vi "NMRvmefull6.vi"() -> ()   [LabVIEW 2013]
uses:
  <vilib>/Utility/file.llb/Read From Spreadsheet File (DBL).vi
  <vilib>/Analysis/NI_AALBase.lvlib
panel:
  out "Telnet error out":errorcluster
  in  "Real/quad Q curve":bool=TRUE
  out "Temperature (C)":dbl(graph)=14.38
  out "+3V supply":dbl=3.03 format="%_4g"
  out "Temp (C)":dbl=14.38 format="%_4g"
  in  "RemovePed":bool=TRUE
  in  "IF / LOG Det":bool
  in  "Q curve file":string="realback213.txt"
  out "File name 2":string="C:\\users\\plm\\Desktop\\rssmt\\realback213.txt"
  in  "AutoBaseline":bool=TRUE
  out "RF OK":bool=TRUE
  out "Peak area (V-MHz)":sgl=0.047433283 format="%.5f"
  in  "Gauss Fit":bool=TRUE
  out "NMR Graph + Fit":cluster{cluster{dbl, "Numeric":dbl}[]}[](graph)=[{[{212.6, "Numeric"=-0.014353571428571417}, {212.60999999999999, "Numeric"=0.00969880952378703}, {212.62, "Numeric"=0.006451190476215146}, {212.63, "Numeric"=0.01930357142857405}, {212.64, "Numeric"=0.0034559523809340603}, {212.65, "Numeric"=0.0017083333333586803}, {212.66, "Numeric"=0.004160714285719118}, {212.67, "Numeric"=-0.02268690476191927}, {212.68, "Numeric"=-0.002834523809498196}, {212.69, "Numeric"=-0.01118214285713618}, {212.7, "Numeric"=0.0006702380952269132}, {212.71, "Numeric"=-0.01337738095235555}, {212.72, "Numeric"=-0.006324999999991986}, {212.73, "Numeric"=-0.0047726190476272586}, {212.74, "Numeric"=-0.0005202380952584774}, {212.75, "Numeric"=-0.0027678571428481173}, {212.76, "Numeric"=-0.009515476190481851}, {212.77, "Numeric"=0.004936904761888499}, {212.78, "Numeric"=-0.01361071428570466}, {212.79, "Numeric"=0.009441666666663164}, {212.8, "Numeric"=-0.0016059523809648993}, {212.81, "Numeric"=0.009946428571438355}, {212.82, "Numeric"=0.011698809523807772}, {212.82999999999998, "Numeric"=0.009451190476178262}, {212.84, "Numeric"=0.0005035714285809706}, {212.85, "Numeric"=-0.013844047619048054}, {212.85999999999999, "Numeric"=0.004308333333324003}, {212.87, "Numeric"=-0.007039285714276826}, {212.88, "Numeric"=0.0008130952380957287}, {212.89, "Numeric"=0.0021654761904693603}, {212.9, "Numeric"=0.007617857142864972}, {212.91, "Numeric"=0.018070238095239086}, {212.92, "Numeric"=0.014822619047614286}, {212.93, "Numeric"=0.03257500000000636}, {212.94, "Numeric"=0.043427380952382036}, {212.95, "Numeric"=0.07847976190475882}, {212.96, "Numeric"=0.12533214285714733}, {212.97, "Numeric"=0.26208452380952457}, {212.98, "Numeric"=0.46923690476190294}, {212.99, "Numeric"=0.47378928571428536}, {213.0, "Numeric"=0.36984166666666674}, {213.01, "Numeric"=0.31639404761904666}, {213.02, "Numeric"=0.28634642857143067}, {213.03, "Numeric"=0.24109880952380847}, {213.04, "Numeric"=0.2555511904761899}, {213.05, "Numeric"=0.2537035714285755}, {213.06, "Numeric"=0.2389559523809498}, {213.07, "Numeric"=0.24110833333333284}, {213.08, "Numeric"=0.20696071428571997}, {213.09, "Numeric"=0.1666130952380907}, {213.1, "Numeric"=0.1359654761904753}, {213.11, "Numeric"=0.105517857142864}, {213.12, "Numeric"=0.0838702380952312}, {213.13, "Numeric"=0.08352261904761737}, {213.14000000000001, "Numeric"=0.06727500000000765}, {213.15, "Numeric"=0.060527380952371285}, {213.16, "Numeric"=0.05027976190475904}, {213.17000000000002, "Numeric"=0.06763214285715088}, {213.18, "Numeric"=0.056484523809510974}, {213.19, "Numeric"=0.010836904761900301}, {213.2, "Numeric"=0.019789285714290707}, {213.21, "Numeric"=-0.0011583333333497411}, {213.22, "Numeric"=0.002394047619041117}, {213.23, "Numeric"=-0.0070535714285668814}, {213.24, "Numeric"=-0.01370119047617081}, {213.25, "Numeric"=-0.01564880952381845}, {213.26, "Numeric"=-0.012996428571424894}, {213.27, "Numeric"=0.002355952380972765}, {213.28, "Numeric"=-0.0036916666666784066}, {213.29, "Numeric"=-0.00803928571428332}, {213.3, "Numeric"=-0.021786904761884066}, {213.31, "Numeric"=-0.007334523809538827}, {213.32, "Numeric"=-0.014282142857142105}, {213.33, "Numeric"=-0.0075297619047413195}, {213.34, "Numeric"=-0.00247738095239957}, {213.35, "Numeric"=-0.01902500000000132}, {213.36, "Numeric"=0.002227380952401034}, {213.37, "Numeric"=-0.0088202380952608}, {213.38, "Numeric"=0.002832142857139036}, {213.39000000000001, "Numeric"=-0.0035154761904570425}, {213.4, "Numeric"=-0.004863095238122388}]}, {[{212.6, "Numeric"=9.804933727167355e-15}, {212.60999999999999, "Numeric"=4.295652004587706e-14}, {212.62, "Numeric"=1.815801447223091e-13}, {212.63, "Numeric"=7.405637705341888e-13}, {212.64, "Numeric"=2.9141466518999593e-12}, {212.65, "Numeric"=1.1064076822601301e-11}, {212.66, "Numeric"=4.0529738278565594e-11}, {212.67, "Numeric"=1.432475667155373e-10}, {212.68, "Numeric"=4.884898512312217e-10}, {212.69, "Numeric"=1.6072323851014186e-09}, {212.7, "Numeric"=5.102190168954913e-09}, {212.71, "Numeric"=1.5627497787480358e-08}, {212.72, "Numeric"=4.6182462698064824e-08}, {212.73, "Numeric"=1.316799241532264e-07}, {212.74, "Numeric"=3.6225708228282077e-07}, {212.75, "Numeric"=9.615437284537467e-07}, {212.76, "Numeric"=2.462498824488131e-06}, {212.77, "Numeric"=6.084681660789618e-06}, {212.78, "Numeric"=1.450622899922786e-05}, {212.79, "Numeric"=3.336768169742033e-05}, {212.8, "Numeric"=7.405465730151238e-05}, {212.81, "Numeric"=0.00015857457517396255}, {212.82, "Numeric"=0.00032761937252901254}, {212.82999999999998, "Numeric"=0.0006530710455585401}, {212.84, "Numeric"=0.00125604766971291}, {212.85, "Numeric"=0.002330808817796288}, {212.85999999999999, "Numeric"=0.004173131021951757}, {212.87, "Numeric"=0.007208953524823476}, {212.88, "Numeric"=0.012015373311762143}, {212.89, "Numeric"=0.019322225631784807}, {212.9, "Numeric"=0.029980016483131332}, {212.91, "Numeric"=0.04488088611738418}, {212.92, "Numeric"=0.0648254911891238}, {212.93, "Numeric"=0.09034103190590272}, {212.94, "Numeric"=0.12147282040713436}, {212.95, "Numeric"=0.15758976979834058}, {212.96, "Numeric"=0.19725670055929137}, {212.97, "Numeric"=0.23822665106036614}, {212.98, "Numeric"=0.27758996627476623}, {212.99, "Numeric"=0.31208437117344906}, {213.0, "Numeric"=0.33852840413966767}, {213.01, "Numeric"=0.35430154417711585}, {213.02, "Numeric"=0.3577715594304534}, {213.03, "Numeric"=0.3485727400272884}, {213.04, "Numeric"=0.3276693836356726}, {213.05, "Numeric"=0.2971892840168628}, {213.06, "Numeric"=0.26006701006465155}, {213.07, "Numeric"=0.21957971714117944}, {213.08, "Numeric"=0.1788767993555635}, {213.09, "Numeric"=0.14059524961771208}, {213.1, "Numeric"=0.10662084409142508}, {213.11, "Numeric"=0.07801325941623595}, {213.12, "Numeric"=0.05507437376443051}, {213.13, "Numeric"=0.03751332412961305}, {213.14000000000001, "Numeric"=0.0246533742775686}, {213.15, "Numeric"=0.015632269227573235}, {213.16, "Numeric"=0.009563624605558374}, {213.17000000000002, "Numeric"=0.005645180762486242}, {213.18, "Numeric"=0.0032150521558659277}, {213.19, "Numeric"=0.0017666602191612085}, {213.2, "Numeric"=0.0009366403752690212}, {213.21, "Numeric"=0.00047912359327834613}, {213.22, "Numeric"=0.00023647055851797608}, {213.23, "Numeric"=0.00011260597483699403}, {213.24, "Numeric"=5.173692702677567e-05}, {213.25, "Numeric"=2.2934784426652083e-05}, {213.26, "Numeric"=9.809424582875055e-06}, {213.27, "Numeric"=4.0480627905257484e-06}, {213.28, "Numeric"=1.6117800860571893e-06}, {213.29, "Numeric"=6.191832059854123e-07}, {213.3, "Numeric"=2.2950248321592862e-07}, {213.31, "Numeric"=8.207491600681828e-08}, {213.32, "Numeric"=2.8319680052242066e-08}, {213.33, "Numeric"=9.428032601552093e-09}, {213.34, "Numeric"=3.0283679848774792e-09}, {213.35, "Numeric"=9.385362566028489e-10}, {213.36, "Numeric"=2.8063917843525365e-10}, {213.37, "Numeric"=8.096557111393358e-11}, {213.38, "Numeric"=2.2537581205675932e-11}, {213.39000000000001, "Numeric"=6.052977548017407e-12}, {213.4, "Numeric"=1.568504102780159e-12}]}]
  in  "Amp of Q curve":dbl=3.0 min=0.0 max=7.0 step=0.01 format="%_3f"
  in  "Subtract Q curve":bool=TRUE
  in  "Adjust Tune":bool
  out "Pedestal Offset":dbl(graph)=-0.0828166666666666
  out "Pedestal Difference":dbl(graph)=-0.05893333333332933
  out "# Good Spectra":i32=988
  in  "Quality cuts":bool=TRUE
  out "Pedestal OK":bool=TRUE
  out "Sweep #":i32=934
  out "1st Sweep":bool
  out "ADC volts OK":bool=TRUE
  out "Peak Height Distribution":cluster{"Y":dbl[], "Y":dbl[]}[](graph)=[{"Y"=[0.35073042256485804, 0.3511598422382979, 0.3515892619117377, 0.3520186815851776, 0.3524481012586174, 0.35287752093205726, 0.3533069406054971, 0.35373636027893696, 0.3541657799523768, 0.35459519962581665, 0.3550246192992565, 0.35545403897269634, 0.3558834586461362, 0.35631287831957603, 0.3567422979930159, 0.3571717176664557, 0.35760113733989557, 0.35803055701333536, 0.3584599766867752, 0.35888939636021505, 0.3593188160336549, 0.35974823570709474, 0.3601776553805346, 0.36060707505397444, 0.3610364947274143, 0.3614659144008541, 0.361895334074294, 0.3623247537477338, 0.36275417342117366, 0.3631835930946135, 0.36361301276805336, 0.3640424324414932, 0.36447185211493305, 0.36490127178837284, 0.3653306914618127, 0.36576011113525253, 0.3661895308086924, 0.3666189504821322, 0.36704837015557207, 0.3674777898290119, 0.36790720950245176, 0.3683366291758916, 0.36876604884933145, 0.3691954685227713, 0.36962488819621114, 0.370054307869651, 0.37048372754309083, 0.3709131472165307, 0.3713425668899705, 0.3717719865634104, 0.37220140623685016, 0.37263082591029, 0.37306024558372985, 0.3734896652571697, 0.37391908493060955, 0.3743485046040494, 0.37477792427748924, 0.3752073439509291, 0.37563676362436893, 0.3760661832978088, 0.3764956029712486, 0.37692502264468847, 0.3773544423181283, 0.37778386199156816, 0.378213281665008, 0.37864270133844785, 0.3790721210118877, 0.3795015406853275, 0.37993096035876733, 0.3803603800322072, 0.380789799705647, 0.38121921937908687, 0.3816486390525267, 0.38207805872596656, 0.3825074783994064, 0.38293689807284625, 0.3833663177462861, 0.38379573741972595, 0.3842251570931658, 0.38465457676660564, 0.3850839964400455, 0.38551341611348533, 0.3859428357869252, 0.38637225546036497, 0.3868016751338048, 0.38723109480724466, 0.3876605144806845, 0.38808993415412435, 0.3885193538275642, 0.38894877350100404, 0.3893781931744439, 0.38980761284788373, 0.3902370325213236, 0.3906664521947634, 0.39109587186820327, 0.3915252915416431, 0.39195471121508296, 0.3923841308885228, 0.39281355056196265, 0.3932429702354025], "Y"=[3.0, 1.0, 2.0, 5.0, 3.0, 2.0, 2.0, 3.0, 2.0, 4.0, 2.0, 5.0, 0.0, 7.0, 1.0, 6.0, 3.0, 2.0, 10.0, 3.0, 4.0, 10.0, 7.0, 4.0, 3.0, 6.0, 6.0, 15.0, 9.0, 15.0, 9.0, 11.0, 13.0, 11.0, 10.0, 17.0, 7.0, 21.0, 15.0, 22.0, 13.0, 22.0, 19.0, 21.0, 18.0, 31.0, 18.0, 20.0, 25.0, 19.0, 16.0, 29.0, 30.0, 17.0, 30.0, 20.0, 19.0, 15.0, 15.0, 10.0, 17.0, 17.0, 18.0, 22.0, 20.0, 10.0, 13.0, 11.0, 13.0, 13.0, 16.0, 3.0, 14.0, 10.0, 12.0, 7.0, 10.0, 8.0, 7.0, 3.0, 9.0, 4.0, 2.0, 3.0, 1.0, 3.0, 4.0, 5.0, 3.0, 1.0, 2.0, 6.0, 3.0, 0.0, 0.0, 5.0, 0.0, 1.0, 0.0, 4.0]}]
  in  "# of Sweeps":i32=1000
  out "Std Dev (V)":dbl=0.008182605348482135 format="%_2g"
  out "Peak mean (V)":dbl=0.37200983179404057 format="%_4g"
  out "Peak Height":dbl(graph)=0.35810372779718896
  in  "Raw Data":bool=TRUE
  in  "Tank RF":bool=TRUE
  in  "IF Atten (dB)":i8 min=0 max=31 step=1
  in  "IFoffset (V)":dbl=-1.9667071999999999 min=-4.0 max=4.0 step=0.001 format="%.4f"
  in  "Tune  (V)":dbl=0.6093999999999999 min=0.0 max=5.0 step=0.001 format="%.4f"
  in  "Hi / Lo IF Gain":bool
  out "Voltage Array":sgl[](array[numeric])=[0.437, 0.436, 0.4083, 0.3973, 0.3582, 0.3338, 0.3142, 0.2659, 0.2649, 0.2363, 0.2285, 0.1954, 0.184, 0.1677, 0.1547, 0.1358, 0.113, 0.112, 0.0786, 0.0874, 0.0627, 0.0612, 0.0505, 0.0364, 0.0162, -0.0088, -0.0007, -0.0215, -0.0225, -0.0294, -0.0316, -0.0282, -0.0379, -0.026, -0.0204, 0.01, 0.0528, 0.1861, 0.3904, 0.3927, 0.2871, 0.2326, 0.2021, 0.157, 0.1722, 0.1717, 0.1589, 0.1636, 0.1326, 0.096, 0.0697, 0.0442, 0.0281, 0.0339, 0.0244, 0.025, 0.0227, 0.0486, 0.0466, 0.0107, 0.03, 0.02, 0.0351, 0.0378, 0.0439, 0.0553, 0.0719, 0.1018, 0.1109, 0.1223, 0.1249, 0.1563, 0.1669, 0.1918, 0.2156, 0.2184, 0.2596, 0.2691, 0.3019, 0.3173, 0.3383] format="%.4f"
  in  "Invert Polarity":bool
  out "Pedestal Diff (V)":sgl=-0.058933333 format="%.3f"
  out "Peak amp (V)":sgl=0.35810372 format="%.3f"
  in  "Save Data to File":bool
  in  "RF Level (dBm)":dbl=-1.0 min=-10.0 max=1.0 step=0.1 format="%.2f"
  out "SMT error out":errorcluster
  out "Sample RMS (V)":dbl=0.011928395061728396 format="%.4f"
  in  "# Sample/step":i32=80 min=1 max=1000 step=100
  in  "Step Width (MHz)":dbl=0.01 min=0.0 max=1000.0 step=0.0005 format="%.4f"
  in  "Freq Span (MHz)":dbl=0.8 min=0.0 max=3000.0 step=0.1 format="%.3f"
  in  "Center Freq (MHz)":dbl=213.0 min=0.005 max=6000.0 step=0.1 format="%.3f"
  in  "Sweep Mode":u16(ring)=3 items=["Off", "Single", "Auto", "Step"]
  in  "GPIB Addr (28)":refnum<visa-resource-name>="GPIB0::28::INSTR"
  # "E1039 Prototype NMR Control Panel"
  # "Settings"
  # "D\nA\nC"
  # "R\nF\n\nG\nE\nN \n\n+\n\nI\nF"
  # "A\nD\nC"
  # "D\nA\nT\nA\n\n+\n\nA \nN\nA\nL\nY\nS\nI\nS"
  # "I\n/\nO"
  # "Results"
  # "A\nv\ne\nr\na\ng\ne"
  # "S\nw\ne\ne\np"
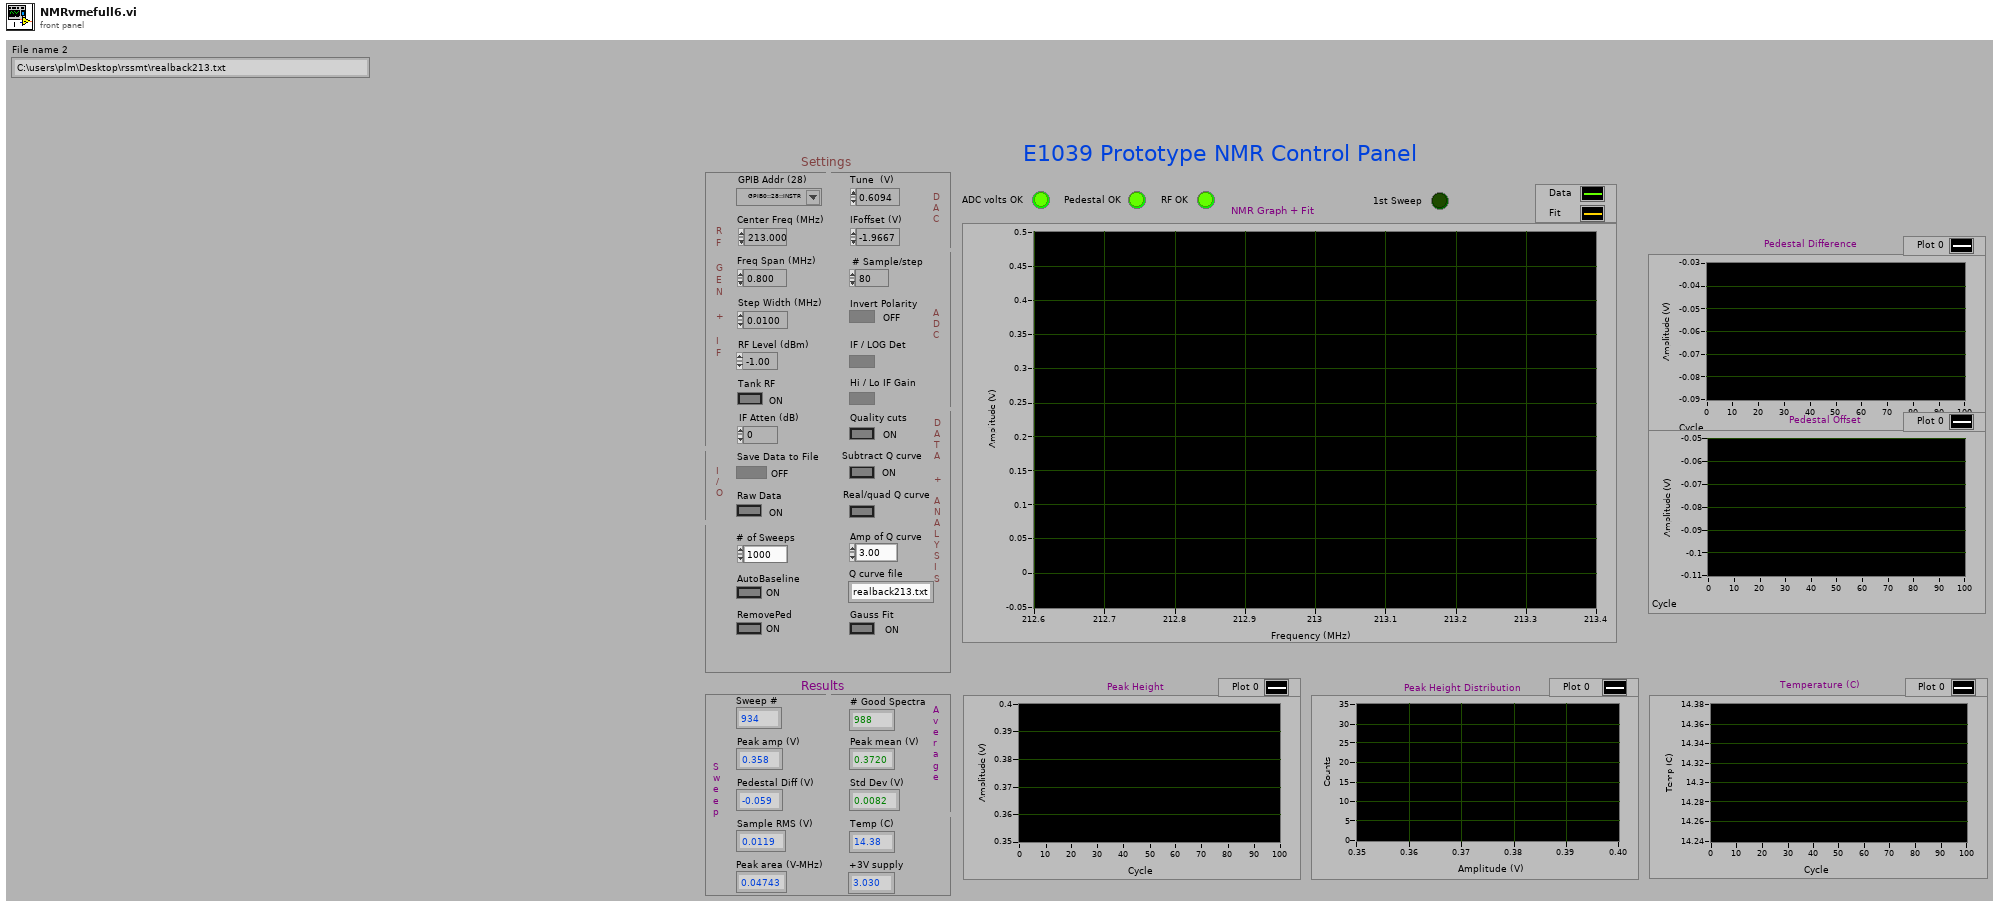
[diagram p1: front panel]
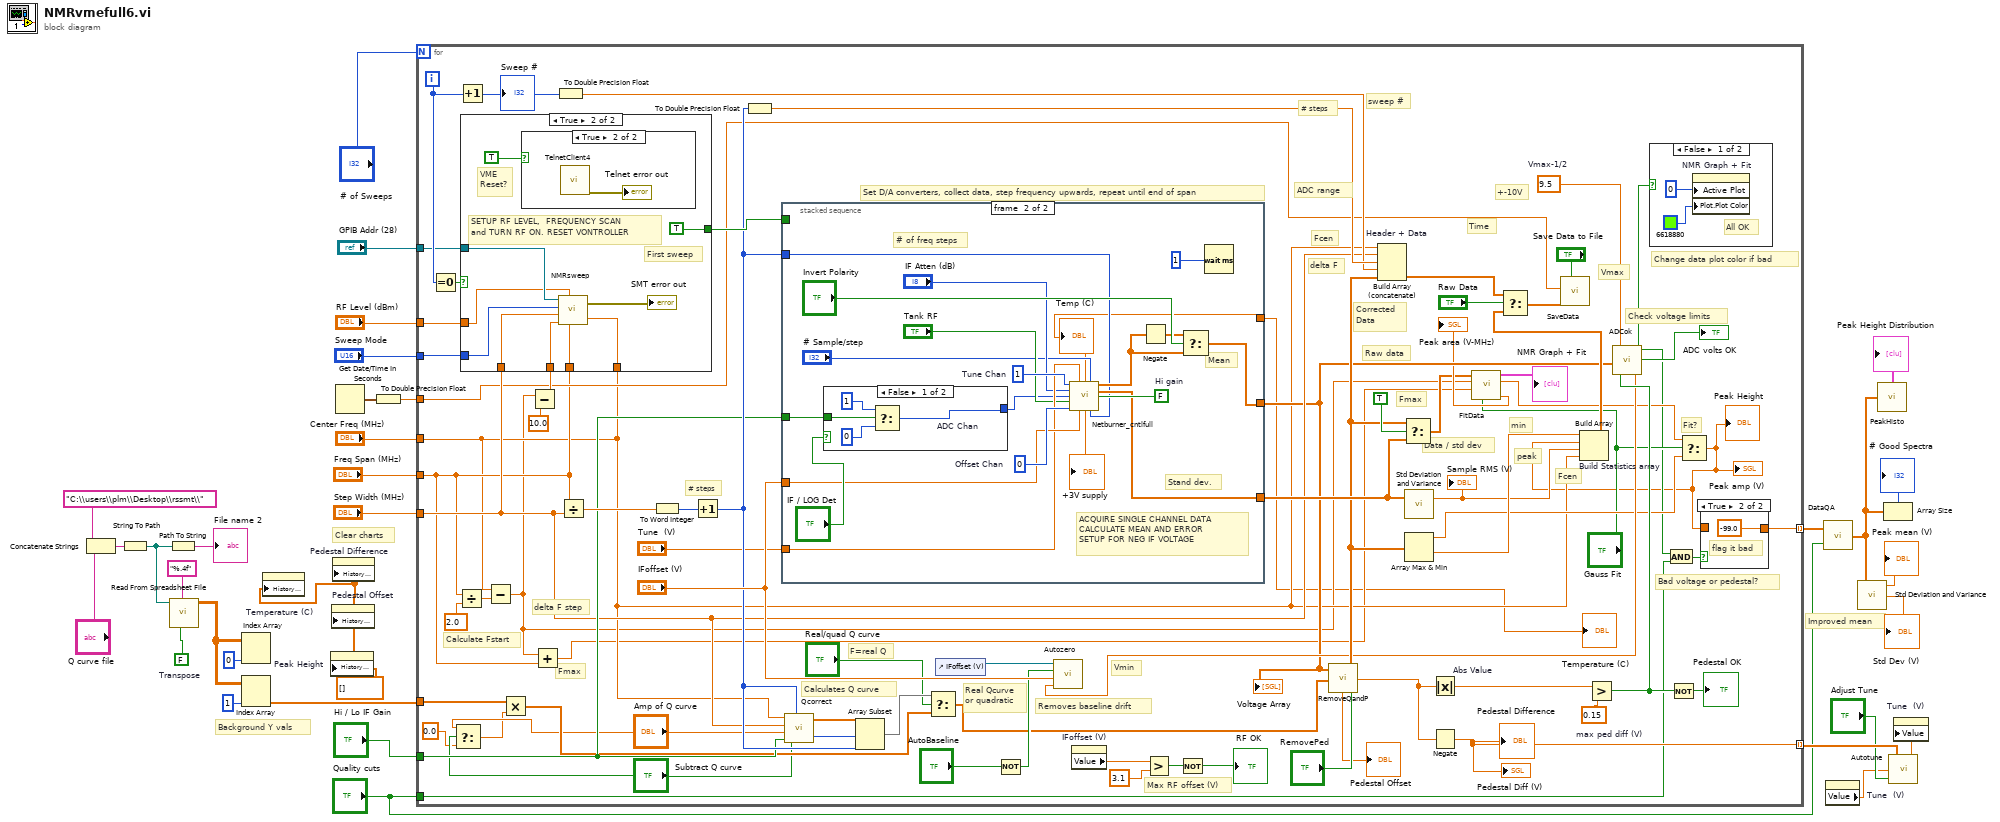
[diagram p0: block diagram]
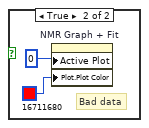
[diagram p2: hidden frame]
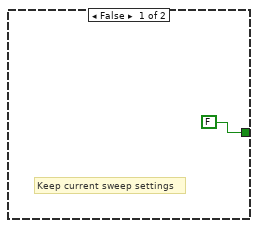
[diagram p4: hidden frame]
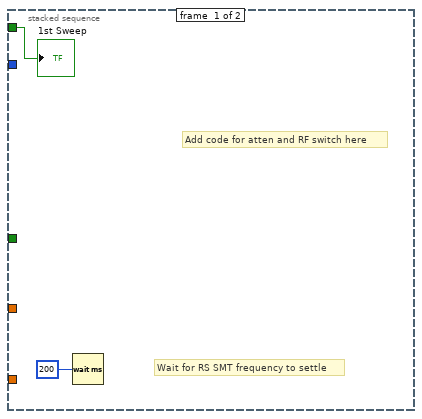
[diagram p6: hidden frame]
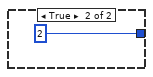
[diagram p7: hidden frame]
diagram:
  w9 = FALSE  # Transpose
  w1 = dbl[] []
  # "Background Y vals"
  # "Clear charts"
  # "Improved mean"
  n1 = Concatenate Strings "Concatenate Strings"("C:\\users\\plm\\Desktop\\rssmt\\", "Q curve file") -> (w12:string)
  n2 = String To Path(string=w12) -> (path=w8:path)
  n3 = Path To String(path=w8) -> (string=→"File name 2":string)
  n4 = call-poly <vilib>:"Read From Spreadsheet File.vi"("transpose (no:F)"=w9, "format (%.3f)"="%.4f", "file path (dialog if empty)"=w8) -> ("all rows"=w7:dbl[][])  [unwired: 4 in, 4 out]
  n5 = Index Array "Index Array"(array=w7, index (col)=0) -> ()  [unwired: 1 in, 1 out]
  n6 = Index Array(array=w7, index (col)=1) -> (element=w2:dbl[])  [unwired: 1 in]
  n7 = property on="Temperature (C)" class="WFChart (strict)"("History Data"=w1) -> ()  [unwired: 2 in, 2 out]
  n8 = property on="Peak Height" class="WFChart (strict)"("History Data"=w1) -> ()  [unwired: 2 in, 2 out]
  n9 = property on="Pedestal Offset" class="WFChart (strict)"("History Data"=w1) -> ()  [unwired: 2 in, 2 out]
  n10 = property on="Pedestal Difference" class="WFChart (strict)"("History Data"=w1) -> ()  [unwired: 2 in, 2 out]
  n11 = Get Date/Time In Seconds() -> (seconds since 1Jan1904=w14:timestamp)
  n12 = To Double Precision Float(number=w14) -> (double precision float=w13:dbl)
  n13 = for {
    N: "# of Sweeps" -> [_]
    tunnel: [w94] -> w29 mode=indexing
    tunnel: "Quality cuts" -> [w71]
    tunnel: [w77] -> w26 mode=indexing
    tunnel: "Center Freq (MHz)" -> [w58]
    tunnel: "Freq Span (MHz)" -> [w64]
    tunnel: "Step Width (MHz)" -> [w70]
    tunnel: "Sweep Mode" -> [w81]
    tunnel: "Hi / Lo IF Gain" -> [w80]
    tunnel: "GPIB Addr (28)" -> [w79]
    tunnel: "RF Level (dBm)" -> [w78]
    tunnel: w13 -> [w65]
    tunnel: w2 -> [w43]
    i -> [w92]
    w75 = 9.5  # Vmax-1/2
    w95 = 0.15  # max ped diff (V)
    # "F=real Q"
    # "Real Qcurve\nor quadratic"
    # "+-10V"
    # "Vmax"
    # "Change data plot color if bad"
    # "Max RF offset (V)"
    # "Fmax"
    # "Fit?"
    # "Fmax"
    # "Time"
    # "Vmin"
    # "min"
    # "peak"
    # "Raw data"
    # "Corrected\nData"
    # "Fcen"
    # "delta F"
    # "# steps"
    # "ADC range"
    # "sweep #"
    # "Fcen"
    # "Set D/A converters, collect data, step frequency upwards, repeat until end of span"
    # "Calculates Q curve"
    # "Removes baseline drift"
    # "Bad voltage or pedestal?"
    # "Check voltage limits"
    # "Data / std dev"
    # "# steps"
    # "Calculate Fstart"
    # "delta F step"
    n14 = Equal To 0?(x=w92) -> (x = 0?=w97:bool)
    n15 = Select(t="Amp of Q curve", s="Subtract Q curve", f=0.0) -> (s? t:f=w38:dbl)
    n16 = Divide(x=w64, y=sgl 2.0) -> (x/y=w108:dbl)
    n17 = Increment(x=w92) -> (x+1=w82:i32)
    "Sweep #" <- w82
    n18 = Subtract(x=w58, y=w108) -> (x-y=w53:dbl)
    n19 = Multiply(x=w43, y=w38) -> (x*y=w42:dbl[])
    n20 = Subtract(x=w53, y=10.0) -> (x-y=w106:dbl)
    n21 = case shown="True" w97 {
      tunnel: w106 -> [_ w127]
      tunnel: w70 -> [_ w125]
      tunnel: w58 -> [_ w124]
      tunnel: w64 -> [_ w126]
      tunnel: [FALSE TRUE] -> w96
      tunnel: w81 -> [_ w121]
      tunnel: w79 -> [_ w120]
      tunnel: w78 -> [_ w119]
      frame False {
        # "Keep current sweep settings"
      }
      frame True {
        # "VME\nReset?"
        # "First sweep"
        # "SETUP RF LEVEL,  FREQUENCY SCAN\nand TURN RF ON. RESET VONTROLLER"
        n22 = case shown="True" TRUE {
          frame False {
          }
          frame True {
            n23 = call "TelnetClient4.vi"() -> ("Telnet error"=→"Telnet error out":errorcluster)  [unwired: 4 in, 3 out]
          }
        }
        n24 = call "NMRsweep.vi"("Center Freq (MHz)"=w124, "Freq Span (MHz)"=w126, "RF Level (dBm)"=w119, "Foffset (MHz)"=w127, "Step Width (MHz)"=w125, "Sweep Mode"=w121, "GPIB Addr (28)"=w120) -> ("error out"=→"SMT error out":errorcluster)
      }
    }
    n25 = Add(x=w53, y=w64) -> (x+y=w52:dbl)
    n26 = To Double Precision Float(number=w82) -> (double precision float=w83:dbl)
    n27 = Divide(x=w64, y=w70) -> (x/y=w110:dbl)
    n28 = To Word Integer(number=w110) -> (16bit integer=w107:i16)
    n29 = Increment(x=w107) -> (x+1=w86:i16)
    n30 = To Double Precision Float(number=w86) -> (double precision float=w85:dbl)
    n31 = stacked-sequence {
      tunnel: [_ w136] -> w100
      tunnel: [_ w148] -> w68
      tunnel: w86 -> [_ w133]
      tunnel: "IFoffset (V)" -> [_ w143]
      tunnel: w80 -> [_ w146]
      tunnel: w96 -> [w129 _]
      tunnel: "Tune  (V)" -> [_ w141]
      tunnel: [_ w131] -> w34
      frame #0 {
        # "Add code for atten and RF switch here"
        # "Wait for RS SMT frequency to settle"
        n32 = Wait (ms)(milliseconds to wait=200) -> ()  [unwired: 1 out]
        "1st Sweep" <- w129
      }
      frame #1 {
        w138 = FALSE  # Hi gain
        w144 = 0  # Offset Chan
        w142 = 1  # Tune Chan
        # "Stand dev."
        # "Mean"
        # "ACQUIRE SINGLE CHANNEL DATA\nCALCULATE MEAN AND ERROR\nSETUP FOR NEG IF VOLTAGE"
        # "# of freq steps"
        n33 = case shown="False" "IF / LOG Det" {
          tunnel: w146 -> [w154 _]
          tunnel: [w151 2] -> w135
          frame False {
            n34 = Select "ADC Chan"(t=1, s=w154, f=0) -> (s? t:f=w151:i32)
          }
          frame True {
          }
        }
        n35 = call "Netburner_cntlfull.vi"("Tune DAC"=w142, "Tune Volt"=w141, "# Data"="# Sample/step", "IF Atten (dB)"="IF Atten (dB)", "NMR ADC"=w135, "Hi Gain"=w138, "Tank RF"="Tank RF", "Offset DAC"=w144, "Offset Volt"=w143, "# f steps"=w133) -> ("Temp (C)"=w131:dbl, "ADC value"=w137:dbl[], "ADC error"=w136:dbl[], "Volts"=→"+3V supply":dbl)  [unwired: 2 out]
        "Temp (C)" <- w131
        n36 = Negate(x=w137) -> (-x=w147:dbl[])
        n37 = Select(t=w147, s="Invert Polarity", f=w137) -> (s? t:f=w148:dbl[])
        n38 = Wait (ms)(milliseconds to wait=1) -> ()  [unwired: 1 out]
      }
    }
    "Voltage Array" <- w68
    "Temperature (C)" <- w34
    n39 = call "Qcorrect.vi"("Subtract Q curve"="Subtract Q curve", "Nstep"=w86, "IF or Log"=w80, "Amp of Q curve"="Amp of Q curve", "Step Width (MHz)"=w70, "Center Freq (MHz)"=w58) -> ("Start"=w101:i32, "Array"=w102:dbl[])
    n40 = Array Subset "Array Subset"(array=w102, index=w101, length=w86) -> (w46:dbl[])
    n41 = Select(t=w46, s="Real/quad Q curve", f=w42) -> (s? t:f=w45:dbl[])
    n42 = control-ref of="IFoffset (V)"() -> (w74:refnum<vi>)
    n43 = Not(x="AutoBaseline") -> (.not. x?=w47:bool)
    n44 = property on="IFoffset (V)" class="DigNum (strict)"() -> ("Value"=w62:dbl)  [unwired: 2 in, 2 out]
    n45 = Greater?(x=w62, y=3.1) -> (0:w60:bool)
    n46 = Not(x=w60) -> (.not. x?=→"RF OK":bool)
    n47 = call "RemoveQandP.vi"("Subtract Ped?"="RemovePed", "Qcurve"=w45, "Raw data"=w68) -> ("Ped L-R"=w88:dbl, "Corrected data"=w84:dbl[], "Ped Offfset"=→"Pedestal Offset":dbl)
    n48 = Build Array (concatenate) "Header + Data"(w58, w70, w85, w83, w84) -> (w87:dbl[])
    n49 = Select(t=w84, s=TRUE, f=w100) -> (s? t:f=w54:dbl[])
    n50 = call <vilib>:"Std Deviation and Variance.vi"("X"=w100) -> ("mean"=w69:dbl)  [unwired: 1 in, 2 out]
    "Sample RMS (V)" <- w69
    n51 = Array Max & Min(array=w84) -> (max value=w63:dbl, min value=w99:dbl)  [unwired: 2 out]
    n52 = Absolute Value "Abs Value"(x=w88) -> (abs(x)=w90:dbl)
    n53 = Negate(x=w88) -> (-x=w77:dbl)
    "Pedestal Diff (V)" <- w77
    "Pedestal Difference" <- w77
    n54 = call "FitData.vi"("Fit?"="Gauss Fit", "Fmax"=w52, "Fmin"=w53, "Yarray"=w54) -> ("Peak Area (V-MHz)"=→"Peak area (V-MHz)":dbl, "Amplitude (V)"=w56:dbl, "NMR Graph + Fit"=→"NMR Graph + Fit":cluster{cluster{dbl, "Numeric":dbl}[]}[])  [unwired: 2 out]
    n55 = Greater?(x=w90, y=w95) -> (0:w76:bool)
    n56 = call "ADCok.vi"("PedOK"=w76, "Array"=w68, "Vmax-1/2"=w75) -> ("Vmin"=w73:dbl, "ADC voltages OK"=→"ADC volts OK":bool, "Allok"=w50:bool)
    n57 = call "Autozero.vi"("Vmin (V)"=w73, "IFoffset (V)"="IFoffset (V)", "IF or Log"=w47, "reference"=w74) -> ()
    n58 = case shown="False" w50 {
      frame False {
        # "All OK"
        n59 = property on="NMR Graph + Fit" class="XYGraph (strict)"("Active Plot"=0, "Plot.Plot Color"=u32 6618880) -> ()  [unwired: 2 in, 2 out]
      }
      frame True {
        # "Bad data"
        n60 = property on="NMR Graph + Fit" class="XYGraph (strict)"("Active Plot"=0, "Plot.Plot Color"=u32 16711680) -> ()  [unwired: 2 in, 2 out]
      }
    }
    n61 = And(x=w50, y=w71) -> (x .and. y?=w91:bool)
    n62 = Not(x=w76) -> (.not. x?=→"Pedestal OK":bool)
    n63 = Select(t=w56, s="Gauss Fit", f=w63) -> (s? t:f=w49:dbl)
    "Peak amp (V)" <- w49
    "Peak Height" <- w49
    n64 = Build Array "Build Statistics array"(w99, w49, w69, w58) -> (w105:dbl[])
    n65 = Select(t=w87, s="Raw Data", f=w105) -> (s? t:f=w66:dbl[])
    n66 = call "SaveData.vi"("Array"=w66, "Save Data to File"="Save Data to File", "Ext time (sec)"=w65) -> ()  [unwired: 1 out]
    n67 = case shown="True" w91 {
      tunnel: [w115 -99.0] -> w94
      tunnel: w49 -> [w115 _]
      frame False {
        # "Data OK"
      }
      frame True {
        # "flag it bad"
      }
    }
  }
  n68 = call "DataQA.vi"("Quality cuts"="Quality cuts", "Data In"=w29) -> ("Data Out"=w28:dbl[])
  n69 = property on="Tune  (V)" class="DigNum (strict)"() -> ("Value"=w17:dbl)  [unwired: 2 in, 2 out]
  n70 = call <vilib>:"Std Deviation and Variance.vi"("X"=w28) -> ("mean"=→"Peak mean (V)":dbl, "standard deviation"=→"Std Dev (V)":dbl)  [unwired: 1 in, 1 out]
  n71 = call "PeakHisto.vi"("Data Out"=w28) -> ("XY Graph"=→"Peak Height Distribution":cluster{"Y":dbl[], "Y":dbl[]}[])
  n72 = Array Size(array=w28) -> (size(s)=→"# Good Spectra":i32)
  n73 = call "Autotune.vi"("Adjust Tune"="Adjust Tune", "Tune Vin"=w17, "Pedestal Diff"=w26) -> ("Tune Vout"=w16:dbl)
  n74 = property on="Tune  (V)" class="DigNum (strict)"("Value"=w16) -> ()  [unwired: 2 in, 2 out]
